vi "GetZipFileFromVI.vi"(2 "New Format?":bool, 3 "VI File":string) -> (0 "Book Name":string, 1 "ZipFile":string)   [LabVIEW 2012]
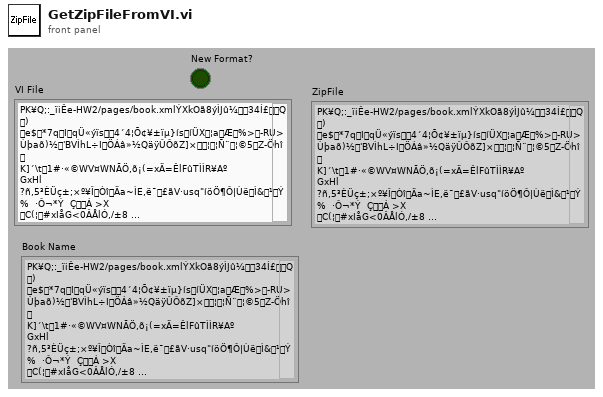
[diagram p1: front panel]
types:
  T1 = enum16{"open", "replace", "create", "open or create", "replace or create", "replace or create with confirmation"}
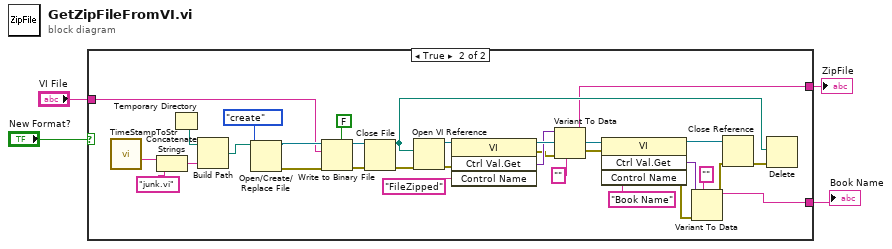
[diagram p0: block diagram]
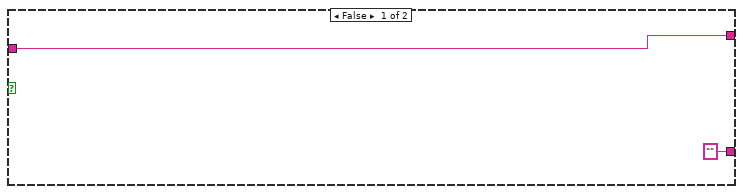
[diagram p2: hidden frame]
diagram:
  n1 = case shown="True" "New Format?" {
    tunnel: "VI File" -> [w6 w28]
    tunnel: [w6 w16] -> w3
    tunnel: ["" ("Control Name") w14] -> w2
    frame False {
    }
    frame True {
      n2 = call <userlib>:"TimeStampToStr.vi"() -> ("date/time string"=w34:string)
      n3 = Concatenate Strings(w34, "junk.vi" ("Remote Path")) -> (w36:string)
      n4 = Temporary Directory() -> (w11:path)
      n5 = Build Path(base path=w11, name or relative path=w36) -> (appended path=w33:path)
      n6 = Open/Create/Replace File(file path (use dialog)=w33, operation (0:open)=T1."create") -> (refnum out=w30:refnum<file>, error out=w29:errorcluster)  [unwired: 1 in, 4 out]
      n7 = Write to Binary File(file (use dialog)=w30, data=w28, error in=w29, 5:FALSE ("prepend array or string size? (T)")) -> (refnum out=w31:refnum<file>, error out=w32:errorcluster)  [unwired: 3 out]
      n8 = Close File(refnum=w31, error in=w32) -> (path=w26:path, error out=w27:errorcluster)
      n9 = Open VI Reference(vi path=w26, error in (no error)=w27) -> (vi reference=w24:refnum<vi>, error out=w25:errorcluster)  [unwired: 4 out]
      n10 = invoke class="VI" method="Ctrl Val.Get"(reference=w24, error in=w25, "Control Name"="FileZipped") -> (reference out=w21:refnum<vi>, error out=w10:errorcluster, "Get Control Value Variant"=w18:variant)  [unwired: 1 in, 1 out]
      n11 = Variant To Data(error in=w10, type="" ("Control Name"), Variant=w18) -> (data=w16:string, error out=w9:errorcluster)
      n12 = invoke class="VI" method="Ctrl Val.Get"(reference=w21, error in=w9, "Control Name"="Book Name") -> (reference out=w20:refnum<vi>, error out=w8:errorcluster, "Get Control Value Variant"=w13:variant)  [unwired: 1 in, 1 out]
      n13 = Variant To Data(error in=w8, type="" ("Control Name"), Variant=w13) -> (data=w14:string, error out=w7:errorcluster)
      n14 = Close Reference(reference=w20, error in (no error)=w7) -> (error out=w23:errorcluster)
      n15 = Delete(path (use dialog)=w26, error in=w23) -> ()  [unwired: 6 out]
    }
  }
  "ZipFile" <- w3
  "Book Name" <- w2
